vi "clone.vi"(0 "reference":refnum<class "AbstractNode.lvclass">, 5 "error in (no error)":errorcluster) -> (14 "reference out":refnum<class "AbstractNode.lvclass">, 15 "clonedAbstractNode":refnum<class "AbstractNode.lvclass">, 19 "error out":errorcluster)   [LabVIEW 2014, in "AbstractNode.lvclass"]
doc: "public Object clone()"
uses:
  <resource>/Framework/Providers/Open_GDS/UML/AbstractNode_class/AbstractNode.lvclass
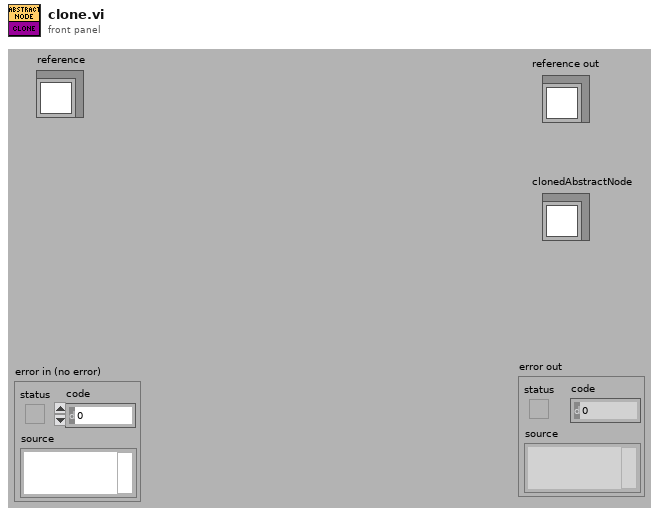
[diagram p1: front panel]
types:
  T1 = typedef "AbstractNode.lvclass/ObjectAttributes.ctl" = cluster{"parent":refnum<class "AbstractNode.lvclass">, "children":refnum<class "AbstractNode.lvclass">[], "Hidden":bool}
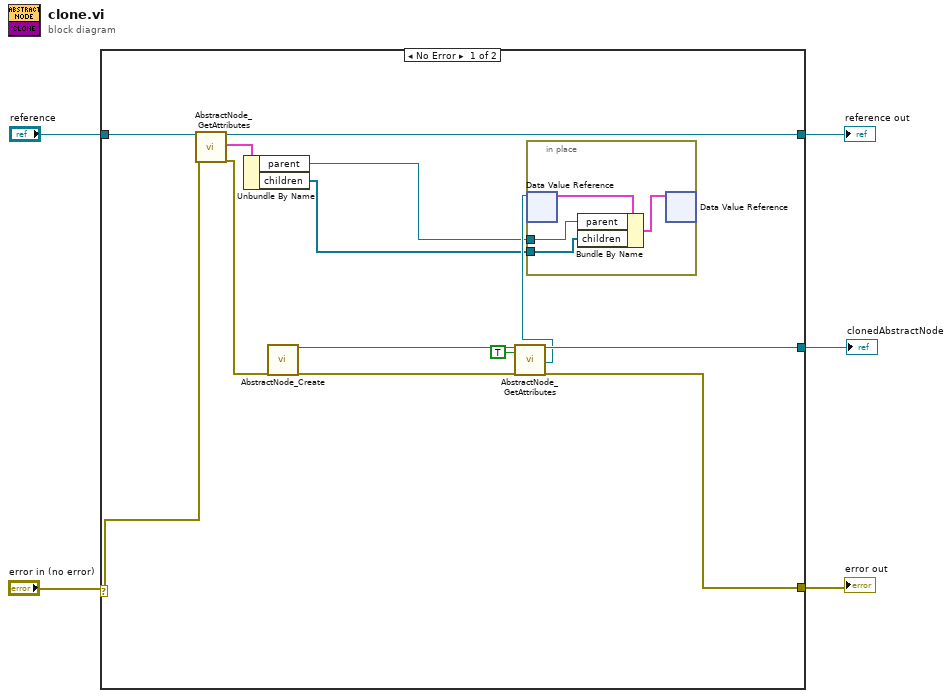
[diagram p0: block diagram]
diagram:
  n1 = case shown="No Error" "error in (no error)" {
    selector: "error in (no error)" -> [w15 w23]
    tunnel: "reference" -> [w18 w24]
    tunnel: [w17 w23] -> w4
    tunnel: [w16 w24] -> w3
    tunnel: [w14 _] -> w1
    frame No Error {
      n2 = call <resource>:"AbstractNode_GetAttributes.vi"("reference in"=w18, "error in (no error)"=w15) -> ("reference out"=w16:refnum<class "AbstractNode.lvclass">, "Data"=w9:T1, "error out"=w11:errorcluster)  [unwired: 1 in, 14 out]
      n3 = Unbundle By Name(w9) -> ("parent"=w7:refnum<class "AbstractNode.lvclass">, "children"=w6:refnum<class "AbstractNode.lvclass">[])
      n4 = call <resource>:"AbstractNode_Create.vi"("error in (no error)"=w11) -> ("reference out"=w13:refnum<class "AbstractNode.lvclass">, "error out"=w12:errorcluster)  [unwired: 1 in, 16 out]
      n5 = call <resource>:"AbstractNode_GetAttributes.vi"("reference in"=w13, "OnlyGetDvrReference(False)"=TRUE, "error in (no error)"=w12) -> ("reference out"=w14:refnum<class "AbstractNode.lvclass">, "DataRef"=w8:refnum<data-value>, "error out"=w17:errorcluster)  [unwired: 13 in, 1 out]
      n6 = in-place {
        in-place-border: w7 -> [w21]
        in-place-border: w6 -> [w20]
        n7 = in-place-dvr #1(w8) -> (w22:T1)  [unwired: 1 out]
        n8 = Bundle By Name(cluster=w22, "parent"=w21, "children"=w20) -> (w19:T1)
        n9 = in-place-dvr #1(w19) -> ()  [unwired: 2 out]
      }
    }
    frame Error {
    }
  }
  "reference out" <- w3
  "error out" <- w4
  "clonedAbstractNode" <- w1
